vi "Read Usb Device Model.vi"(8 "error in (no error)":errorcluster) -> (0 "error out":errorcluster, 3 "Return":u32)   [LabVIEW 2010, in "TPVG_DLL.lvlib"]
doc: "This function must be called to read device model\n\n---------------------------------------------------------------\nWritten by: Dang Lam"
uses:
  TPVG_DLL.lvlib
  TPVG_DLL.dll
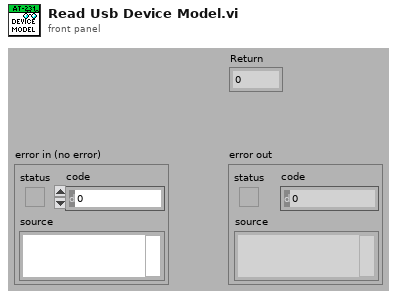
[diagram p1: front panel]
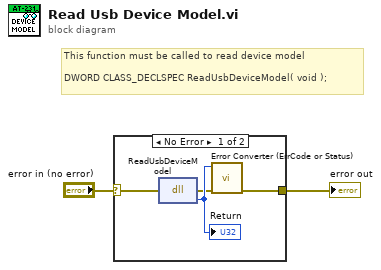
[diagram p0: block diagram]
diagram:
  # "This function must be called to read device model\n\nDWORD CLASS_DECLSPEC ReadUsbDeviceModel( void );"
  n1 = case shown="No Error" "error in (no error)" {
    selector: "error in (no error)" -> [w3 w7]
    tunnel: [w4 w7] -> w2
    frame No Error {
      n2 = dll-call lib="TPVG_DLL.dll" fn="ReadUsbDeviceModel"(error in=w3) -> (error out=w5:errorcluster, "return type"=w6:u32)  [unwired: 2 in, 1 out]
      "Return" <- w6
      n3 = call "Error Converter (ErrCode or Status).vi"("error in (no error)"=w5, "error code"=w6) -> ("error out"=w4:errorcluster)  [unwired: 9 in]
    }
    frame Error {
    }
  }
  "error out" <- w2
